vi "Picture_shr_Save_to_matlab.vi"   [LabVIEW 2011]
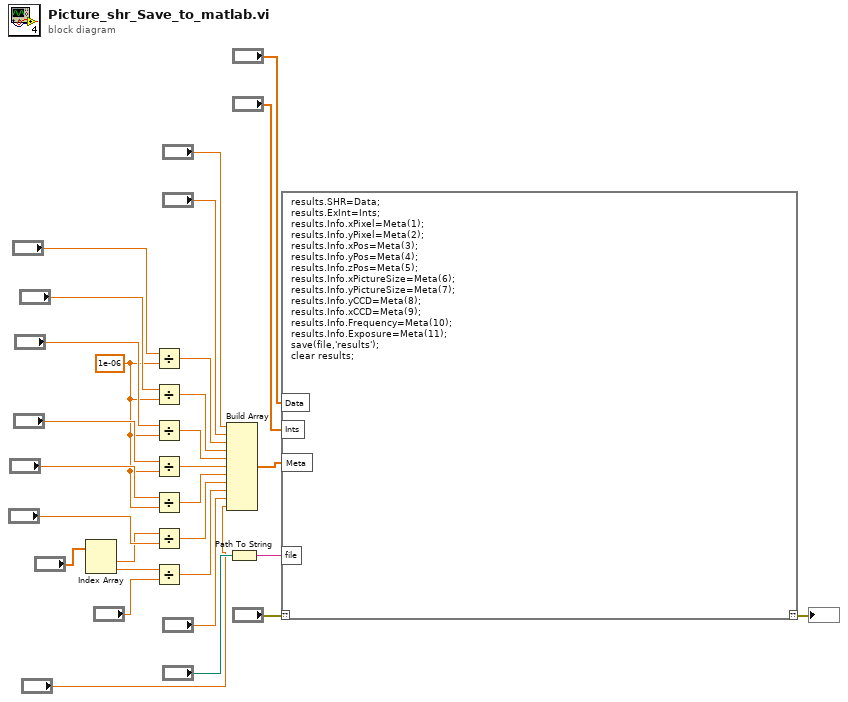
[diagram p0: block diagram]
diagram:
  w8 = 1e-06 ("y")
  n1 = Index Array(array="?") -> (element #1=w3:dbl, element #2=w4:dbl)  [unwired: 2 in]
  n2 = Divide(x="?", y=w8) -> (x/y=w21:dbl)
  n3 = Divide(x="?", y=w8) -> (x/y=w20:dbl)
  n4 = Divide(x="?", y=w8) -> (x/y=w23:dbl)
  n5 = Divide(x="?", y=w8) -> (x/y=w22:dbl)
  n6 = Divide(x="?", y=w8) -> (x/y=w24:dbl)
  n7 = Divide(x=w3, y="?") -> (x/y=w25:dbl)
  n8 = Divide(x=w4, y="?") -> (x/y=w26:dbl)
  n9 = Build Array("?", "?", w21, w20, w23, w22, w24, w25, w26, "?", "?") -> (w27:dbl[])
  n10 = Path To String(path="?") -> (string=w28:string)
  n11 = script code="results.SHR=Data;\nresults.ExInt=Ints;\nresults.Info.xPixel=Meta(1);\nresults.Info.yPixel=Meta(2);\nresults.Info.xPos=Meta(3);\nresults.Info.yPos=Meta(4);\nresults.Info.zPos=Meta(5);\nresults.Info.xPictureSize=Meta(6);\nresults.Info.yPictureSize=Meta(7);\nresults.Info.yCCD=Meta(8);\nresults.Info.xCCD=Meta(9);\nresults.Info.Frequency=Meta(10);\nresults.Info.Exposure=Meta(11);\nsave(file,'results');\nclear results;"("??"="?", "Data"="?", "Ints"="?", "Meta"=w27, "file"=w28) -> ("??"=→"?":errorcluster)
